vi "Connect.vi"(7 "Address":string, 8 "error in":errorcluster, 9 "ICommHandler in":refnum<class "ICommHandler.lvclass">) -> (2 "error out":errorcluster, 3 "ICommHandler out":refnum<class "ICommHandler.lvclass">)   [LabVIEW 2020, in "wamplv.lvlib" / "ICommHandler.lvclass"]
uses:
  <userlib>/wamplv/Comm Handlers/ICommHandler/ICommHandler.lvclass
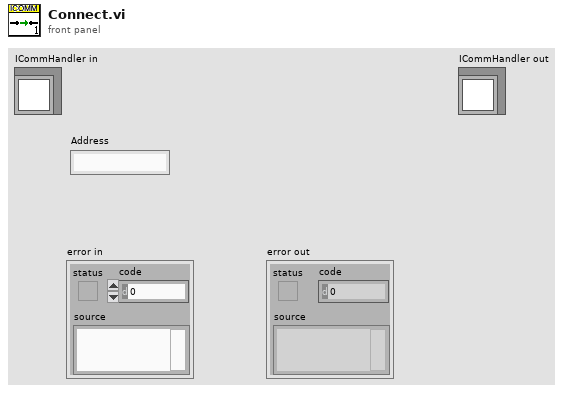
[diagram p1: front panel]
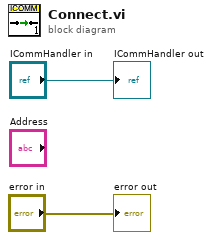
[diagram p0: block diagram]
diagram:
  "ICommHandler out" <- "ICommHandler in"
  "error out" <- "error in"
